vi "SetSenseResistor.vi"(6 "Set Button":bool, 7 "Sense Resistor":u32, 8 "error in":errorcluster, 9 "Previous Channel":string, 10 "PastScalingFactor":dbl, 11 "VISA resource name":refnum<visa-resource-name>) -> (0 "error out 2":errorcluster, 1 "Current Channel":string, 2 "CurrentScalingFactor":dbl, 3 "VISA resource name out":refnum<visa-resource-name>, 4 "isCorrect":bool)   [LabVIEW 2012]
panel:
  out "read string":string
  out "bytes read":u32
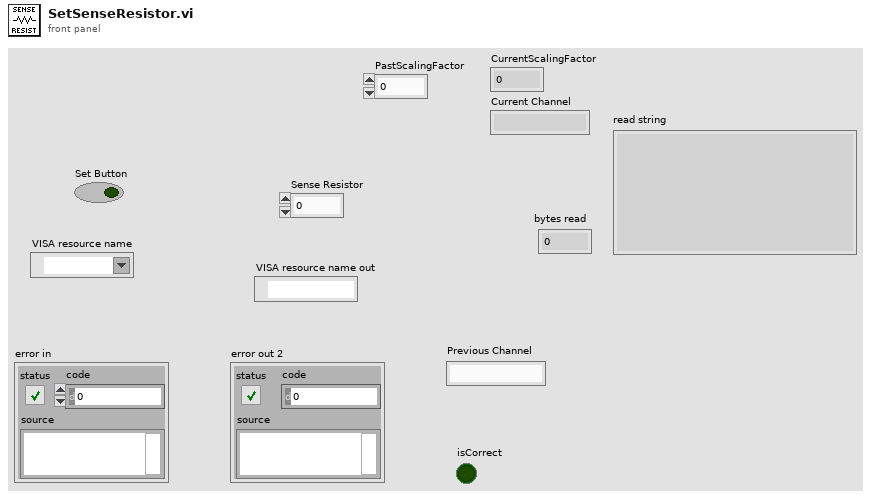
[diagram p1: front panel]
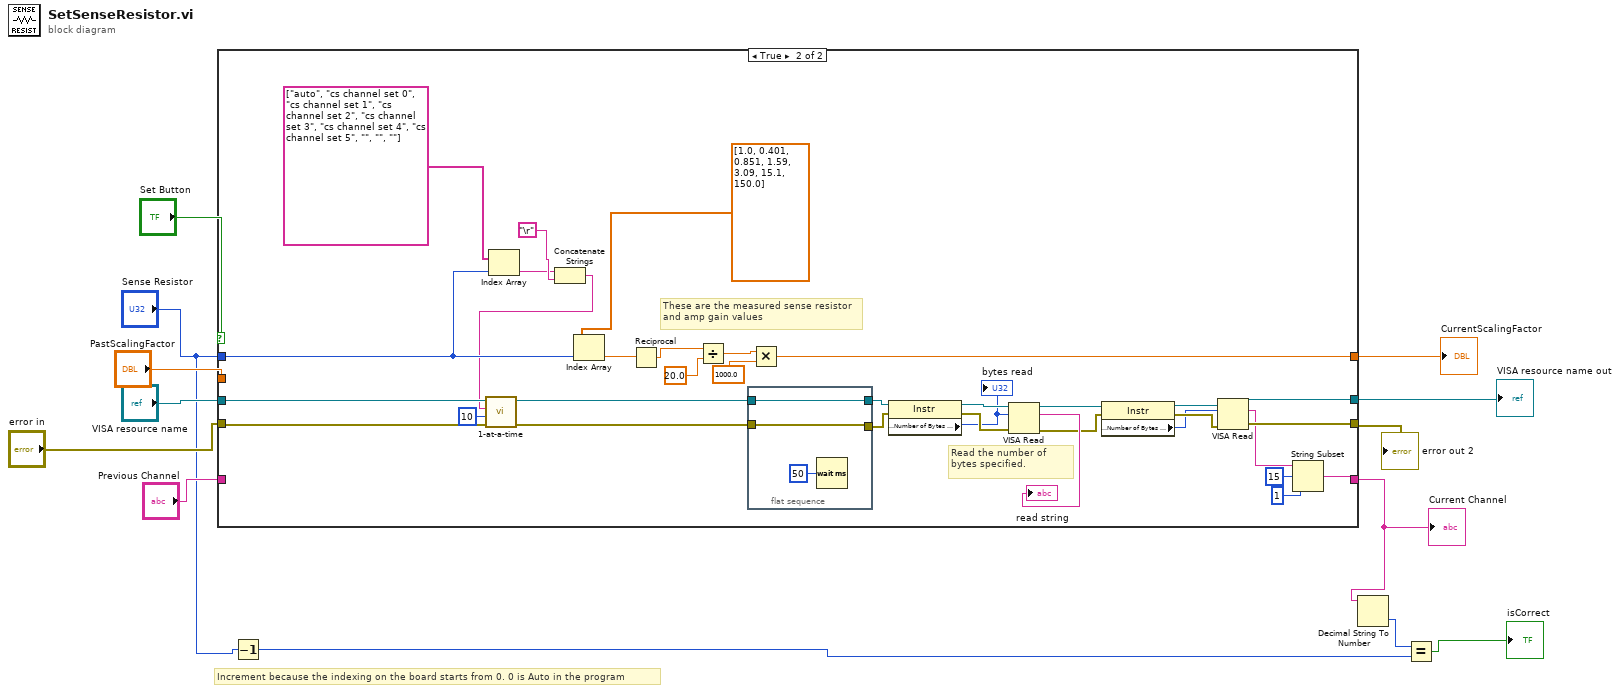
[diagram p0: block diagram]
diagram:
  # "Increment because the indexing on the board starts from 0. 0 is Auto in the program"
  n1 = case shown="True" "Set Button" {
    tunnel: "VISA resource name" -> [w17 w51]
    tunnel: "error in" -> [w16 w50]
    tunnel: [w17 w31] -> w8
    tunnel: [w16 w30] -> w9
    tunnel: "Sense Resistor" -> [_ w39]
    tunnel: [w15 w37] -> w13
    tunnel: "PastScalingFactor" -> [w15 _]
    tunnel: [w14 w20] -> w5
    tunnel: "Previous Channel" -> [w14 _]
    frame False {
    }
    frame True {
      # "Read the number of bytes specified."
      # "These are the measured sense resistor\nand amp gain values"
      n2 = Index Array(array=string[] ["auto", "cs channel set 0", "cs channel set 1", "cs channel set 2", "cs channel set 3", "cs channel set 4", "cs channel set 5", "", "", ""], index=w39) -> (element=w41:string)
      n3 = Concatenate Strings(w41, "\r") -> (w38:string)
      n4 = call "1-at-a-time.vi"("error in (no error)"=w50, "Wait Between Characters(ms)"=u32 10, "write buffer"=w38, "VISA resource name"=w51) -> ("error out"=w27:errorcluster, "VISA resource name out"=w28:refnum<visa-resource-name>)  [unwired: 5 in, 1 out]
      n5 = Index Array(array=dbl[] [1.0, 0.401, 0.851, 1.59, 3.09, 15.1, 150.0], index=w39) -> (element=w47:dbl)
      n6 = Reciprocal(x=w47) -> (1/x=w46:dbl)
      n7 = Divide(x=w46, y=20.0 ("x")) -> (x/y=w43:dbl)
      n8 = flat-sequence {
        tunnel: [w54] -> w33
        tunnel: w28 -> [w54]
        tunnel: [w53] -> w32
        tunnel: w27 -> [w53]
        frame #0 {
          n9 = Wait (ms)(milliseconds to wait=u32 50) -> ()  [unwired: 1 out]
        }
      }
      n10 = Multiply(x=w43, y=1000.0) -> (x*y=w37:dbl)
      n11 = property class="Instr"(reference=w33, error in=w32) -> (reference out=w36:refnum<visa-resource-name>, error out=w35:errorcluster, "Serial Settings:Number of Bytes at Serial Port"=w29:u32)
      "bytes read" <- w29
      n12 = VISA Read(VISA resource name=w36, byte count=w29, error in (no error)=w35) -> (VISA resource name out=w26:refnum<visa-resource-name>, read buffer=→"read string":string, error out=w25:errorcluster)  [unwired: 1 out]
      n13 = property class="Instr"(reference=w26, error in=w25) -> (reference out=w24:refnum<visa-resource-name>, error out=w23:errorcluster, "Serial Settings:Number of Bytes at Serial Port"=w22:u32)
      n14 = VISA Read(VISA resource name=w24, byte count=w22, error in (no error)=w23) -> (VISA resource name out=w31:refnum<visa-resource-name>, read buffer=w21:string, error out=w30:errorcluster)  [unwired: 1 out]
      n15 = String Subset(string=w21, offset (0)=15, length (rest)=1 ("length (rest)")) -> (substring=w20:string)
    }
  }
  "CurrentScalingFactor" <- w13
  "error out 2" <- w9
  "VISA resource name out" <- w8
  "Current Channel" <- w5
  n16 = Decrement(x="Sense Resistor") -> (x-1=w1:u32)
  n17 = Decimal String To Number(string=w5) -> (number=w4:i32)  [unwired: 2 in, 1 out]
  n18 = Equal?(x=w4, y=w1) -> (x = y?=→"isCorrect":bool)
